vi "log analysis_gps.vi"() -> ()   [LabVIEW 2018] (continued)
\t\n15:44:38.5\tlog_raw\tgps_raw\t\tsystem status\tnormal 2 27.900000 0 0\trobot status\t150.631494\t124.442843\t7.927600\t-0.100159\t-0.498264\t-179.473329\t0.268000\t-0.011000\n\t\n15:44:39.0\tlog_raw\tgps_raw\t\tsystem status\tnormal 2 27.900000 0 0\trobot status\t150.478452\t124.453463\t7.927100\t-0.269341\t-0.623918\t-179.511393\t0.246000\t0.046000\n\t\n15:44:39.5\tlog_raw\tgps_raw\t\tsystem status\tnormal 2 27.900000 0 0\trobot status\t150.333282\t124.462585\t7.928600\t-0.322841\t-0.681958\t-179.469049\t0.260000\t0.066000\n\t\n15:44:40.0\tlog_raw\tgps_raw\t\tsystem status\tnormal 2 27.900000 0 0\trobot status\t150.188702\t124.473109\t7.929800\t-0.268389\t-0.694858\t-179.390159\t0.304000\t0.005000\n\t\n15:44:40.5\tlog_raw\tgps_raw\t\tsystem status\tnormal 2 27.800000 0 0\trobot status\t150.046673\t124.482305\t7.929800\t-0.234085\t-0.771225\t-179.316552\t0.299000\t0.006000\n\t\n15:44:41.0\tlog_raw\tgps_raw\t\tsystem status\tnormal 2 27.900000 0 0\trobot status\t149.902023\t124.492124\t7.930600\t-0.171880\t-0.860108\t-179.202739\t0.268000\t0.042000\n\t\n15:44:41.5\tlog_raw\tgps_raw\t\tsystem status\tnormal 2 27.800000 0 0\trobot status\t149.758940\t124.501657\t7.931700\t-0.049577\t-0.856104\t-179.098606\t0.422000\t-0.186000\n\t\n15:44:42.0\tlog_raw\tgps_raw\t#INSPVAXA,USB3,0,49.5,FINESTEERING,2107,283500.050,02000000,471d,15824;INS_ALIGNMENT_COMPLETE,INS_RTKFIXED,37.37125208894,126.72252418884,7.9323,22.3000,0.0457,-0.3130,0.0162,0.019884592,-0.737230354,268.941103131,0.4422,0.2953,0.5719,0.1133,0.0925,0.0782,0.0964,0.1015,5.0570,0f000001,0*24f2188e\n\tsystem status\tnormal 2 27.800000 0 0\trobot status\t149.616272\t124.511447\t7.932300\t0.019885\t-0.737230\t-178.941103\t0.282000\t0.036000\n\t\n15:44:42.5\tlog_raw\tgps_raw\t\tsystem status\tnormal 2 27.900000 0 0\trobot status\t149.500042\t124.520050\t7.931800\t0.135214\t-0.708677\t-178.779585\t0.109000\t0.043000\n\t\n15:44:43.0\tlog_raw\tgps_raw\t\tsystem status\tnormal 2 27.900000 0 0\trobot status\t149.355950\t124.527273\t7.930800\t0.129535\t-0.692129\t-178.620902\t0.232000\t0.079000\n\t\n15:44:43.5\tlog_raw\tgps_raw\t\tsystem status\tnormal 2 27.900000 0 0\trobot status\t149.217281\t124.534073\t7.930700\t0.247819\t-0.669048\t-178.512392\t0.338000\t-0.027000\n\t\n15:44:44.1\tlog_raw\tgps_raw\t\tsystem status\tnormal 2 27.900000 0 0\trobot status\t149.075473\t124.540045\t7.931300\t0.217256\t-0.509981\t-178.436963\t0.306000\t0.005000\n\t\n15:44:44.6\tlog_raw\tgps_raw\t\tsystem status\tnormal 2 27.800000 0 0\trobot status\t148.934943\t124.543786\t7.931500\t0.099168\t-0.402207\t-178.296990\t0.326000\t-0.034000\n\t\n15:44:45.1\tlog_raw\tgps_raw\t\tsystem status\tnormal 2 27.800000 0 0\trobot status\t148.793897\t124.549425\t7.932200\t0.131171\t-0.388845\t-178.227976\t0.263000\t0.053000\n\t\n15:44:45.6\tlog_raw\tgps_raw\t\tsystem status\tnormal 2 27.900000 0 0\trobot status\t148.653222\t124.555022\t7.931500\t0.252835\t-0.357965\t-178.170042\t0.368000\t-0.106000\n\t\n15:44:46.1\tlog_raw\tgps_raw\t\tsystem status\tnormal 2 27.900000 0 0\trobot status\t148.511244\t124.560395\t7.931600\t0.240454\t-0.345271\t-178.148997\t0.365000\t-0.109000\n\t\n15:44:46.6\tlog_raw\tgps_raw\t\tsystem status\tnormal 2 27.800000 0 0\trobot status\t148.370007\t124.561874\t7.933900\t-0.038867\t-0.502153\t-178.139470\t0.289000\t0.017000\n\t\n15:44:47.1\tlog_raw\tgps_raw\t\tsystem status\tnormal 2 27.900000 0 0\trobot status\t148.234752\t124.565255\t7.935600\t-0.119013\t-0.587133\t-178.082740\t0.262000\t-0.016000\n\t\n15:44:47.6\tlog_raw\tgps_raw\t\tsystem status\tnormal 2 27.800000 0 0\trobot status\t148.145131\t124.569753\t7.937200\t-0.177448\t-0.292844\t-177.902896\t0.342000\t0.062000\n\t\n15:44:48.1\tlog_raw\tgps_raw\t\tsystem status\tnormal 2 27.900000 0 0\trobot status\t148.008420\t124.573995\t7.938300\t-0.006356\t-0.091938\t-177.926561\t0.275000\t-0.003000\n\t\n15:44:48.6\tlog_raw\tgps_raw\t\tsystem status\tnormal 2 27.900000 0 0\trobot status\t147.862293\t124.576815\t7.938300\t0.010797\t-0.019689\t-178.073343\t0.278000\t0.019000\n\t\n15:44:49.1\tlog_raw\tgps_raw\t\tsystem status\tnormal 2 27.900000 0 0\trobot status\t147.729188\t124.580815\t7.939000\t-0.029685\t0.130111\t-178.108993\t0.304000\t-0.009000\n\t\n15:44:49.6\tlog_raw\tgps_raw\t\tsystem status\tnormal 2 27.900000 0 0\trobot status\t147.592276\t124.583432\t7.941800\t-0.099788\t0.170966\t-178.169157\t0.309000\t-0.006000\n\t\n15:44:50.1\tlog_raw\tgps_raw\t#INSPVAXA,USB3,0,48.5,FINESTEERING,2107,283508.100,02000000,471d,15824;INS_ALIGNMENT_COMPLETE,INS_RTKFIXED,37.37125276901,126.72249960907,7.9453,22.3000,0.0373,-0.2902,0.0053,-0.191217202,-0.027683345,268.229043523,0.4412,0.2949,0.5722,0.1131,0.0925,0.0782,0.0964,0.1013,5.0646,0f000001,0*8b85f82b\n\tsystem status\tnormal 2 27.900000 0 0\trobot status\t147.439036\t124.586963\t7.945300\t-0.191217\t-0.027683\t-178.229044\t0.301000\t-0.004000\n\t\n15:44:50.6\tlog_raw\tgps_raw\t\tsystem status\tnormal 2 27.900000 0 0\trobot status\t147.313297\t124.590519\t7.946400\t-0.139869\t-0.013929\t-178.296761\t0.298000\t-0.006000\n\t\n15:44:51.1\tlog_raw\tgps_raw\t#INSPVAXA,USB3,0,51.0,FINESTEERING,2107,283509.100,02000000,471d,15824;INS_ALIGNMENT_COMPLETE,INS_RTKFIXED,37.37125284410,126.72249644466,7.9470,22.3000,0.0401,-0.2879,-0.0045,-0.106806668,-0.162103067,268.404823616,0.4419,0.2950,0.5723,0.1130,0.0925,0.0782,0.0964,0.1013,5.0643,0f000001,0*7bfc8e45\n\tsystem status\tnormal 2 27.900000 0 0\trobot status\t147.158738\t124.595302\t7.947000\t-0.106807\t-0.162103\t-178.404824\t0.301000\t-0.004000\n\t\n15:44:51.6\tlog_raw\tgps_raw\t\tsystem status\tnormal 2 27.900000 0 0\trobot status\t147.032825\t124.599819\t7.947800\t-0.058595\t-0.300497\t-178.519340\t0.302000\t-0.003000\n\t\n15:44:52.1\tlog_raw\tgps_raw\t\tsystem status\tnormal 2 27.900000 0 0\trobot status\t146.935693\t124.606222\t7.947200\t0.018402\t-0.342096\t-178.435886\t0.265000\t-0.053000\n\t\n15:44:52.6\tlog_raw\tgps_raw\t\tsystem status\tnormal 2 27.900000 0 0\trobot status\t146.775595\t124.607523\t7.947200\t-0.117241\t-0.394741\t-178.589413\t0.321000\t-0.041000\n\t\n15:44:53.1\tlog_raw\tgps_raw\t#INSPVAXA,USB3,0,49.5,FINESTEERING,2107,283511.100,02000000,471d,15824;INS_ALIGNMENT_COMPLETE,INS_RTKFIXED,37.37125297857,126.72249062368,7.9478,22.3000,0.0268,-0.2671,0.0078,-0.192910717,-0.348782343,268.576521671,0.4435,0.2952,0.5725,0.1132,0.0925,0.0782,0.0964,0.1012,5.0632,0f000001,0*b468220b\n\tsystem status\tnormal 2 27.900000 0 0\trobot status\t146.643125\t124.610235\t7.947800\t-0.192911\t-0.348782\t-178.576522\t0.289000\t-0.019000\n\t\n15:44:53.6\tlog_raw\tgps_raw\t\tsystem status\tnormal 2 27.900000 0 0\trobot status\t146.501637\t124.614064\t7.947700\t-0.071913\t-0.322697\t-178.749577\t0.298000\t-0.007000\n\t\n15:44:54.1\tlog_raw\tgps_raw\t#INSPVAXA,USB3,0,46.5,FINESTEERING,2107,283512.100,02000000,471d,15824;INS_ALIGNMENT_COMPLETE,INS_RTKFIXED,37.37125304820,126.72248734658,7.9477,22.3000,0.0144,-0.2984,0.0121,-0.146751568,-0.096737224,268.816557460,0.4452,0.2954,0.5727,0.1133,0.0925,0.0782,0.0964,0.1013,5.0625,0f000001,0*292499ae\n\tsystem status\tnormal 2 27.900000 0 0\trobot status\t146.352845\t124.617968\t7.947700\t-0.146752\t-0.096737\t-178.816557\t0.306000\t0.006000\n\t\n15:44:54.6\tlog_raw\tgps_raw\t#INSPVAXA,USB3,0,46.5,FINESTEERING,2107,283512.600,02000000,471d,15824;INS_ALIGNMENT_COMPLETE,INS_RTKFIXED,37.37125307400,126.72248575305,7.9480,22.3000,0.0122,-0.2749,0.0049,-0.358672753,0.036676838,268.917809450,0.4452,0.2954,0.5727,0.1133,0.0925,0.0782,0.0964,0.1013,5.0625,0f000001,0*09269caa\n\tsystem status\tnormal 2 27.900000 0 0\trobot status\t146.211692\t124.620834\t7.948000\t-0.358673\t0.036677\t-178.917809\t0.296000\t-0.004000\n\t\n15:44:55.1\tlog_raw\tgps_raw\t\tsystem status\tnormal 2 27.900000 0 0\trobot status\t146.080792\t124.623760\t7.947900\t-0.500734\t0.107504\t-179.034616\t0.296000\t-0.003000\n\t\n15:44:55.6\tlog_raw\tgps_raw\t\tsystem status\tnormal 2 27.900000 0 0\trobot status\t145.941875\t124.628534\t7.948000\t-0.533837\t0.131507\t-179.099176\t0.299000\t0.000000\n\t\n15:44:56.1\tlog_raw\tgps_raw\t\tsystem status\tnormal 2 27.900000 0 0\trobot status\t145.802261\t124.634287\t7.948900\t-0.548226\t0.140549\t-179.167826\t0.300000\t-0.002000\n\t\n15:44:56.6\tlog_raw\tgps_raw\t\tsystem status\tnormal 2 27.900000 0 0\trobot status\t145.663385\t124.642656\t7.949000\t-0.592979\t-0.128506\t-179.213932\t0.148000\t0.018000\n\t\n15:44:57.1\tlog_raw\tgps_raw\t\tsystem status\tnormal 2 27.800000 0 0\trobot status\t145.577746\t124.651687\t7.948600\t-0.583585\t-0.125120\t-179.114339\t0.350000\t0.047000\n\t\n15:44:57.6\tlog_raw\tgps_raw\t\tsystem status\tnormal 2 27.900000 0 0\trobot status\t145.399589\t124.657796\t7.947700\t-0.657699\t-0.498657\t-179.343167\t0.272000\t0.019000\n\t\n15:44:58.1\tlog_raw\tgps_raw\t#INSPVAXA,USB3,0,46.0,FINESTEERING,2107,283516.100,02000000,471d,15824;INS_ALIGNMENT_COMPLETE,INS_RTKFIXED,37.37125347923,126.72247506393,7.9472,22.3000,0.0170,-0.3545,-0.0054,-0.698217493,-0.526151709,269.397858351,0.4451,0.2957,0.5732,0.1136,0.0925,0.0782,0.0963,0.1013,5.0659,0f000001,0*b20fee82\n\tsystem status\tnormal 2 27.800000 0 0\trobot status\t145.264868\t124.665825\t7.947200\t-0.698217\t-0.526152\t-179.397858\t0.311000\t0.015000\n\t\n15:44:58.6\tlog_raw\tgps_raw\t\tsystem status\tnormal 2 27.900000 0 0\trobot status\t145.120868\t124.672886\t7.946700\t-0.698968\t-0.760852\t-179.547331\t0.292000\t0.004000\n\t\n15:44:59.1\tlog_raw\tgps_raw\t#INSPVAXA,USB3,0,52.0,FINESTEERING,2107,283517.100,02000000,471d,15824;INS_ALIGNMENT_COMPLETE,INS_RTKFIXED,37.37125363028,126.72247167466,7.9449,22.3000,0.0243,-0.3135,0.0010,-0.686347073,-0.797841284,269.600362862,0.4443,0.2956,0.5732,0.1135,0.0925,0.0782,0.0963,0.1013,5.0669,0f000001,0*80e32c69\n\tsystem status\tnormal 2 27.900000 0 0\trobot status\t144.964652\t124.682594\t7.944900\t-0.686347\t-0.797841\t-179.600363\t0.315000\t0.000000\n\t\n15:44:59.6\tlog_raw\tgps_raw\t\tsystem status\tnormal 2 27.900000 0 0\trobot status\t144.838880\t124.691376\t7.944400\t-0.566112\t-0.739210\t-179.635847\t0.288000\t-0.001000\n\t\n15:45:00.1\tlog_raw\tgps_raw\t\tsystem status\tnormal 2 27.900000 0 0\trobot status\t144.692090\t124.700615\t7.944700\t-0.547013\t-0.597270\t-179.727134\t0.296000\t0.005000\n\t\n15:45:00.6\tlog_raw\tgps_raw\t#INSPVAXA,USB3,0,49.0,FINESTEERING,2107,283518.600,02000000,471d,15824;INS_ALIGNMENT_COMPLETE,INS_RTKFIXED,37.37125389857,126.72246679519,7.9445,22.3000,0.0331,-0.3036,0.0138,-0.450567847,-0.447424519,269.738401914,0.4438,0.2956,0.5732,0.1134,0.0925,0.0782,0.0963,0.1013,5.0679,0f000001,0*e0521a7f\n\tsystem status\tnormal 2 27.900000 0 0\trobot status\t144.532436\t124.712378\t7.944500\t-0.450568\t-0.447425\t-179.738402\t0.306000\t0.009000\n\t\n15:45:01.1\tlog_raw\tgps_raw\t\tsystem status\tnormal 2 27.900000 0 0\trobot status\t144.402361\t124.721254\t7.944400\t-0.605900\t-0.247307\t-179.812526\t0.286000\t-0.015000\n\t\n15:45:01.6\tlog_raw\tgps_raw\t\tsystem status\tnormal 2 27.800000 0 0\trobot status\t144.307793\t124.732072\t7.945200\t-0.557084\t-0.001971\t-179.605860\t0.321000\t0.030000\n\t\n15:45:02.1\tlog_raw\tgps_raw\t#INSPVAXA,USB3,0,48.0,FINESTEERING,2107,283520.100,02000000,471d,15824;INS_ALIGNMENT_COMPLETE,INS_RTKFIXED,37.37125419691,126.72246226393,7.9458,22.3000,0.0272,-0.1971,0.0083,-0.453121577,-0.197375891,269.782721447,0.4440,0.2956,0.5733,0.1137,0.0925,0.0782,0.0963,0.1013,5.0706,0f000001,0*56a37df9\n\tsystem status\tnormal 2 27.900000 0 0\trobot status\t144.131065\t124.745496\t7.945800\t-0.453122\t-0.197376\t-179.782721\t0.241000\t0.083000\n\t\n15:45:02.6\tlog_raw\tgps_raw\t#INSPVAXA,USB3,0,51.0,FINESTEERING,2107,283520.600,02000000,471d,15824;INS_ALIGNMENT_COMPLETE,INS_RTKFIXED,37.37125430556,126.72246059927,7.9481,22.3000,0.0288,-0.2781,0.0031,-0.463416060,-0.290924424,269.736679663,0.4440,0.2956,0.5733,0.1137,0.0925,0.0782,0.0963,0.1013,5.0706,0f000001,0*484206e1\n\tsystem status\tnormal 2 27.900000 0 0\trobot status\t143.983612\t124.757557\t7.948100\t-0.463416\t-0.290924\t-179.736680\t0.260000\t0.074000\n\t\n15:45:03.1\tlog_raw\tgps_raw\t\tsystem status\tnormal 2 27.800000 0 0\trobot status\t143.858446\t124.769127\t7.950000\t-0.373602\t-0.343041\t-179.624970\t0.393000\t-0.117000\n\t\n15:45:03.6\tlog_raw\tgps_raw\t\tsystem status\tnormal 2 27.900000 0 0\trobot status\t143.714422\t124.779252\t7.952600\t-0.516012\t-0.390078\t-179.534175\t0.262000\t0.064000\n\t\n15:45:04.1\tlog_raw\tgps_raw\t#INSPVAXA,USB3,0,50.0,FINESTEERING,2107,283522.100,02000000,471d,15824;INS_ALIGNMENT_COMPLETE,INS_RTKFIXED,37.37125461142,126.72245575598,7.9554,22.3000,0.0322,-0.2902,-0.0060,-0.575699494,-0.254956238,269.403721782,0.4439,0.2957,0.5734,0.1134,0.0925,0.0782,0.0963,0.1013,5.0736,0f000001,0*4d3ff4ec\n\tsystem status\tnormal 2 27.800000 0 0\trobot status\t143.554601\t124.791510\t7.955400\t-0.575699\t-0.254956\t-179.403722\t0.286000\t0.027000\n\t\n15:45:04.6\tlog_raw\tgps_raw\t#INSPVAXA,USB3,0,50.0,FINESTEERING,2107,283522.600,02000000,471d,15824;INS_ALIGNMENT_COMPLETE,INS_RTKFIXED,37.37125471396,126.72245415918,7.9561,22.3000,0.0355,-0.2916,-0.0127,-0.527584053,-0.253715800,269.126606548,0.4439,0.2957,0.5734,0.1134,0.0925,0.0782,0.0963,0.1013,5.0736,0f000001,0*ec5fc995\n\tsystem status\tnormal 2 27.800000 0 0\trobot status\t143.413159\t124.802893\t7.956100\t-0.527584\t-0.253716\t-179.126607\t0.295000\t0.016000\n\t\n15:45:05.1\tlog_raw\tgps_raw\t#INSPVAXA,USB3,0,48.5,FINESTEERING,2107,283523.100,02000000,471d,15824;INS_ALIGNMENT_COMPLETE,INS_RTKFIXED,37.37125482190,126.72245252510,7.9566,22.3000,0.0302,-0.2961,-0.0010,-0.338922460,-0.418464715,268.895183147,0.4433,0.2957,0.5734,0.1134,0.0926,0.0782,0.0963,0.1013,5.0752,0f000001,0*1d6fb429\n\tsystem status\tnormal 2 27.800000 0 0\trobot status\t143.268415\t124.814875\t7.956600\t-0.338922\t-0.418465\t-178.895183\t0.302000\t0.007000\n\t\n15:45:05.6\tlog_raw\tgps_raw\t#INSPVAXA,USB3,0,48.5,FINESTEERING,2107,283523.600,02000000,471d,15824;INS_ALIGNMENT_COMPLETE,INS_RTKFIXED,37.37125490537,126.72245090226,7.9573,22.3000,0.0299,-0.3022,0.0033,-0.516635552,-0.400593547,268.699996239,0.4433,0.2957,0.5734,0.1134,0.0926,0.0782,0.0963,0.1013,5.0752,0f000001,0*027b4151\n\tsystem status\tnormal 2 27.800000 0 0\trobot status\t143.124666\t124.824141\t7.957300\t-0.516636\t-0.400594\t-178.699996\t0.373000\t-0.101000\n\t\n15:45:06.1\tlog_raw\tgps_raw\t#INSPVAXA,USB3,0,49.5,FINESTEERING,2107,283524.100,02000000,471d,15824;INS_ALIGNMENT_COMPLETE,INS_RTKFIXED,37.37125498193,126.72244929891,7.9584,22.3000,0.0403,-0.2922,0.0032,-0.646627486,-0.365479151,268.410156940,0.4428,0.2959,0.5733,0.1133,0.0925,0.0782,0.0963,0.1013,5.0766,0f000001,0*7811970f\n\tsystem status\tnormal 2 27.800000 0 0\trobot status\t142.982644\t124.832640\t7.958400\t-0.646627\t-0.365479\t-178.410157\t0.376000\t-0.111000\n\t\n15:45:06.6\tlog_raw\tgps_raw\t\tsystem status\tnormal 2 27.800000 0 0\trobot status\t142.855371\t124.839702\t7.959100\t-0.637911\t-0.389706\t-178.125788\t0.419000\t-0.171000\n\t\n15:45:07.1\tlog_raw\tgps_raw\t\tsystem status\tnormal 2 27.800000 0 0\trobot status\t142.714130\t124.849046\t7.959500\t-0.466492\t-0.305331\t-177.961176\t0.297000\t0.007000\n\t\n15:45:07.6\tlog_raw\tgps_raw\t#INSPVAXA,USB3,0,47.5,FINESTEERING,2107,283525.600,02000000,471d,15824;INS_ALIGNMENT_COMPLETE,INS_RTKFIXED,37.37125519906,126.72244452104,7.9610,22.3000,0.0264,-0.2896,0.0115,-0.459568698,-0.292533166,267.670803857,0.4424,0.2958,0.5732,0.1133,0.0925,0.0782,0.0963,0.1013,5.0781,0f000001,0*17724b4e\n\tsystem status\tnormal 2 27.800000 0 0\trobot status\t142.559428\t124.856746\t7.961000\t-0.459569\t-0.292533\t-177.670804\t0.405000\t-0.152000\n\t\n15:45:08.1\tlog_raw\tgps_raw\t#INSPVAXA,USB3,0,47.0,FINESTEERING,2107,283526.100,02008000,471d,15824;INS_ALIGNMENT_COMPLETE,INS_RTKFIXED,37.37125524446,126.72244292133,7.9621,22.3000,0.0343,-0.2757,0.0102,-0.752609295,-0.423876797,267.522844293,0.4423,0.2959,0.5731,0.1133,0.0925,0.0782,0.0963,0.1013,5.0795,0f000001,0*e02a1c85\n\tsystem status\tnormal 2 27.800000 0 0\trobot status\t142.417729\t124.861787\t7.962100\t-0.752609\t-0.423877\t-177.522844\t0.227000\t0.100000\n\t\n15:45:08.6\tlog_raw\tgps_raw\t\tsystem status\tnormal 2 27.800000 0 0\trobot status\t142.289996\t124.866450\t7.964000\t-0.891263\t-0.489713\t-177.486596\t0.339000\t-0.052000\n\t\n15:45:09.1\tlog_raw\tgps_raw\t#INSPVAXA,USB3,0,47.0,FINESTEERING,2107,283527.100,02008000,471d,15824;INS_ALIGNMENT_COMPLETE,INS_RTKFIXED,37.37125535577,126.72243973319,7.9657,22.3000,0.0385,-0.2807,-0.0002,-0.916031014,-0.466994988,267.419817945,0.4418,0.2957,0.5731,0.1132,0.0925,0.0782,0.0963,0.1013,5.0811,0f000001,0*de1342cb\n\tsystem status\tnormal 2 27.900000 0 0\trobot status\t142.135329\t124.874145\t7.965700\t-0.916031\t-0.466995\t-177.419818\t0.306000\t-0.017000\n\t\n15:45:09.6\tlog_raw\tgps_raw\t#INSPVAXA,USB3,0,48.0,FINESTEERING,2107,283527.600,02008000,471d,15824;INS_ALIGNMENT_COMPLETE,INS_RTKFIXED,37.37125539878,126.72243810634,7.9658,22.3000,0.0326,-0.2757,-0.0036,-1.071635503,-0.660283197,267.417863682,0.4418,0.2957,0.5731,0.1132,0.0925,0.0782,0.0963,0.1013,5.0811,0f000001,0*715093d1\n\tsystem status\tnormal 2 27.900000 0 0\trobot status\t141.991225\t124.878921\t7.965800\t-1.071636\t-0.660283\t-177.417864\t0.236000\t0.079000\n\t\n15:45:10.1\tlog_raw\tgps_raw\t#INSPVAXA,USB3,0,46.5,FINESTEERING,2107,283528.100,02008000,471d,15824;INS_ALIGNMENT_COMPLETE,INS_RTKFIXED,37.37125544077,126.72243647488,7.9658,22.3000,0.0284,-0.2919,-0.0061,-1.262244823,-0.886371740,267.477769914,0.4412,0.2955,0.5730,0.1131,0.0925,0.0782,0.0963,0.1013,5.0826,0f000001,0*a5d2d267\n\tsystem status\tnormal 2 27.900000 0 0\trobot status\t141.846713\t124.883584\t7.965800\t-1.262245\t-0.886372\t-177.477770\t0.371000\t-0.108000\n\t\n15:45:10.6\tlog_raw\tgps_raw\t\tsystem status\tnormal 2 27.900000 0 0\trobot status\t141.737271\t124.888134\t7.965800\t-1.358773\t-1.011232\t-177.503415\t0.249000\t-0.023000\n\t\n15:45:11.1\tlog_raw\tgps_raw\t#INSPVAXA,USB3,0,51.5,FINESTEERING,2107,283529.100,02008000,471d,15824;INS_ALIGNMENT_COMPLETE,INS_RTKFIXED,37.37125551038,126.72243332814,7.9661,22.3000,0.0230,-0.2496,0.0003,-1.593217414,-1.364879356,267.511520433,0.4406,0.2953,0.5729,0.1132,0.0926,0.0782,0.0963,0.1012,5.0841,0f000001,0*c5d25f23\n\tsystem status\tnormal 2 27.900000 0 0\trobot status\t141.567980\t124.891314\t7.966100\t-1.593217\t-1.364879\t-177.511520\t0.254000\t0.059000\n\t\n15:45:11.6\tlog_raw\tgps_raw\t#INSPVAXA,USB3,0,51.5,FINESTEERING,2107,283529.600,02008000,471d,15824;INS_ALIGNMENT_COMPLETE,INS_RTKFIXED,37.37125553545,126.72243179074,7.9678,22.3000,0.0177,-0.3268,0.0196,-1.900322132,-1.296600351,267.646844528,0.4406,0.2953,0.5729,0.1132,0.0926,0.0782,0.0963,0.1012,5.0841,0f000001,0*bf0a8b51\n\tsystem status\tnormal 2 27.900000 0 0\trobot status\t141.431799\t124.894099\t7.967800\t-1.900322\t-1.296600\t-177.646845\t0.334000\t-0.025000\n\t\n15:45:12.1\tlog_raw\tgps_raw\t#INSPVAXA,USB3,0,51.0,FINESTEERING,2107,283530.100,02008000,471d,15824;INS_ALIGNMENT_COMPLETE,INS_RTKFIXED,37.37125556979,126.72243022543,7.9689,22.3000,0.0347,-0.2712,0.0165,-2.106253221,-1.191638715,267.711415615,0.4397,0.2950,0.5729,0.1130,0.0929,0.0782,0.0963,0.1012,5.0852,0f000001,0*30fd5459\n\tsystem status\tnormal 2 27.900000 0 0\trobot status\t141.293147\t124.897913\t7.968900\t-2.106253\t-1.191639\t-177.711416\t0.278000\t0.006000\n\t\n15:45:12.6\tlog_raw\tgps_raw\t#INSPVAXA,USB3,0,51.0,FINESTEERING,2107,283530.600,02000000,471d,15824;INS_ALIGNMENT_COMPLETE,INS_RTKFIXED,37.37125561825,126.72242855799,7.9691,22.3000,0.0407,-0.2688,0.0120,-2.213736166,-1.038882938,267.844151397,0.4397,0.2950,0.5729,0.1130,0.0929,0.0782,0.0963,0.1012,5.0852,0f000001,0*ed713259\n\tsystem status\tnormal 2 27.900000 0 0\trobot status\t141.145448\t124.903293\t7.969100\t-2.213736\t-1.038883\t-177.844151\t0.287000\t0.006000\n\t\n15:45:13.1\tlog_raw\tgps_raw\t#INSPVAXA,USB3,0,43.5,FINESTEERING,2107,283531.100,02000000,471d,15824;INS_ALIGNMENT_COMPLETE,INS_RTKFIXED,37.37125567803,126.72242699713,7.9701,22.3000,0.0384,-0.2967,0.0169,-2.258821559,-0.728124735,267.962573337,0.4398,0.2947,0.5728,0.1130,0.0928,0.0782,0.0963,0.1012,5.0855,0f000001,0*96bde39a\n\tsystem status\tnormal 2 27.900000 0 0\trobot status\t141.007189\t124.909930\t7.970100\t-2.258822\t-0.728125\t-177.962573\t0.307000\t-0.007000\n\t\n15:45:13.6\tlog_raw\tgps_raw\t#INSPVAXA,USB3,0,43.5,FINESTEERING,2107,283531.600,02000000,471d,15824;INS_ALIGNMENT_COMPLETE,INS_RTKFIXED,37.37125573053,126.72242543109,7.9712,22.3000,0.0393,-0.2946,0.0161,-2.393557008,-0.508805819,268.092577363,0.4398,0.2947,0.5728,0.1130,0.0928,0.0782,0.0963,0.1012,5.0855,0f000001,0*fb176aea\n\tsystem status\tnormal 2 27.900000 0 0\trobot status\t140.868472\t124.915759\t7.971200\t-2.393557\t-0.508806\t-178.092577\t0.301000\t-0.006000\n\t\n15:45:14.1\tlog_raw\tgps_raw\t\tsystem status\tnormal 2 27.900000 0 0\trobot status\t140.736365\t124.922041\t7.972000\t-2.497682\t-0.394077\t-178.262431\t0.297000\t-0.011000\n\t\n15:45:14.6\tlog_raw\tgps_raw\t#INSPVAXA,USB3,0,46.5,FINESTEERING,2107,283532.600,02000000,471d,15824;INS_ALIGNMENT_COMPLETE,INS_RTKFIXED,37.37125585668,126.72242215627,7.9725,22.3000,0.0380,-0.3002,0.0167,-2.444436463,-0.411927002,268.408506598,0.4408,0.2948,0.5728,0.1133,0.0928,0.0782,0.0963,0.1013,5.0851,0f000001,0*752f38e5\n\tsystem status\tnormal 2 27.900000 0 0\trobot status\t140.578394\t124.929765\t7.972500\t-2.444436\t-0.411927\t-178.408507\t0.303000\t-0.003000\n\t\n15:45:15.1\tlog_raw\tgps_raw\t#INSPVAXA,USB3,0,46.5,FINESTEERING,2107,283533.100,02000000,471d,15824;INS_ALIGNMENT_COMPLETE,INS_RTKFIXED,37.37125592571,126.72242055610,7.9738,22.3000,0.0424,-0.2920,0.0172,-2.420399044,-0.549310631,268.532317727,0.4414,0.2948,0.5728,0.1132,0.0926,0.0782,0.0963,0.1012,5.0840,0f000001,0*330bd1f6\n\tsystem status\tnormal 2 27.900000 0 0\trobot status\t140.436653\t124.937429\t7.973800\t-2.420399\t-0.549311\t-178.532318\t0.296000\t-0.007000\n\t\n15:45:15.6\tlog_raw\tgps_raw\t#INSPVAXA,USB3,0,49.5,FINESTEERING,2107,283533.600,02000000,471d,15824;INS_ALIGNMENT_COMPLETE,INS_RTKFIXED,37.37125599617,126.72241909319,7.9758,22.3000,0.0239,-0.2932,0.0057,-2.389135000,-0.690009705,268.630043000,0.4414,0.2948,0.5728,0.1132,0.0926,0.0782,0.0963,0.1012,5.0840,0f000001,0*946e4f45\n\tsystem status\tnormal 2 27.900000 0 0\trobot status\t140.307071\t124.945251\t7.975800\t-2.389135\t-0.690010\t-178.630043\t0.283000\t-0.023000\n\t\n15:45:16.1\tlog_raw\tgps_raw\t#INSPVAXA,USB3,0,46.5,FINESTEERING,2107,283534.100,02000000,471d,15824;INS_ALIGNMENT_COMPLETE,INS_RTKFIXED,37.37125606459,126.72241729161,7.9768,22.3000,0.0318,-0.3014,0.0051,-2.433419723,-0.928712698,268.813892776,0.4412,0.2949,0.5728,0.1131,0.0925,0.0782,0.0963,0.1012,5.0833,0f000001,0*8f6d80c9\n\tsystem status\tnormal 2 27.900000 0 0\trobot status\t140.147490\t124.952847\t7.976800\t-2.433420\t-0.928713\t-178.813893\t0.294000\t-0.008000\n\t\n15:45:16.6\tlog_raw\tgps_raw\t#INSPVAXA,USB3,0,46.5,FINESTEERING,2107,283534.600,02000000,471d,15824;INS_ALIGNMENT_COMPLETE,INS_RTKFIXED,37.37125615079,126.72241575292,7.9767,22.3000,0.0422,-0.2723,0.0071,-2.318351029,-0.994572866,268.928791382,0.4412,0.2949,0.5728,0.1131,0.0925,0.0782,0.0963,0.1012,5.0833,0f000001,0*09e2fdbf\n\tsystem status\tnormal 2 27.900000 0 0\trobot status\t140.011195\t124.962416\t7.976700\t-2.318351\t-0.994573\t-178.928791\t0.294000\t-0.011000\n\t\n15:45:17.1\tlog_raw\tgps_raw\t#INSPVAXA,USB3,0,46.5,FINESTEERING,2107,283535.100,02000000,471d,15824;INS_ALIGNMENT_COMPLETE,INS_RTKFIXED,37.37125625866,126.72241406717,7.9767,22.3000,0.0424,-0.2966,-0.0053,-2.021295828,-1.106669357,269.086555595,0.4405,0.2950,0.5729,0.1131,0.0926,0.0782,0.0963,0.1012,5.0840,0f000001,0*6efa0b45\n\tsystem status\tnormal 2 27.900000 0 0\trobot status\t139.861874\t124.974391\t7.976700\t-2.021296\t-1.106669\t-179.086556\t0.304000\t-0.001000\n\t\n15:45:17.6\tlog_raw\tgps_raw\t#INSPVAXA,USB3,0,46.5,FINESTEERING,2107,283535.600,02000000,471d,15824;INS_ALIGNMENT_COMPLETE,INS_RTKFIXED,37.37125636363,126.72241247006,7.9775,22.3000,0.0475,-0.2765,0.0068,-1.865554802,-1.007723760,269.206912297,0.4405,0.2950,0.5729,0.1131,0.0926,0.0782,0.0963,0.1012,5.0840,0f000001,0*0c6af5d6\n\tsystem status\tnormal 2 27.900000 0 0\trobot status\t139.720405\t124.986043\t7.977500\t-1.865555\t-1.007724\t-179.206912\t0.298000\t-0.006000\n\t\n15:45:18.1\tlog_raw\tgps_raw\t#INSPVAXA,USB3,0,47.5,FINESTEERING,2107,283536.100,02000000,471d,15824;INS_ALIGNMENT_COMPLETE,INS_RTKFIXED,37.37125647369,126.72241083113,7.9788,22.3000,0.0521,-0.3007,0.0049,-1.790943231,-0.806222731,269.320889615,0.4398,0.2953,0.5729,0.1129,0.0928,0.0782,0.0963,0.1012,5.0856,0f000001,0*d4e8effb\n\tsystem status\tnormal 2 27.900000 0 0\trobot status\t139.575231\t124.998260\t7.978800\t-1.790943\t-0.806223\t-179.320890\t0.302000\t0.001000\n\t\n15:45:18.6\tlog_raw\tgps_raw\t#INSPVAXA,USB3,0,47.5,FINESTEERING,2107,283536.600,02000000,471d,15824;INS_ALIGNMENT_COMPLETE,INS_RTKFIXED,37.37125658130,126.72240921238,7.9784,22.3000,0.0588,-0.2967,0.0032,-1.856879731,-0.578836067,269.400871435,0.4398,0.2953,0.5729,0.1129,0.0928,0.0782,0.0963,0.1012,5.0856,0f000001,0*690b56d4\n\tsystem status\tnormal 2 27.900000 0 0\trobot status\t139.431845\t125.010206\t7.978400\t-1.856880\t-0.578836\t-179.400871\t0.302000\t0.001000\n\t\n15:45:19.1\tlog_raw\tgps_raw\t#INSPVAXA,USB3,0,46.0,FINESTEERING,2107,283537.100,02000000,471d,15824;INS_ALIGNMENT_COMPLETE,INS_RTKFIXED,37.37125671293,126.72240759051,7.9784,22.3000,0.0622,-0.2885,0.0100,-1.691821646,-0.334147317,269.491731881,0.4392,0.2956,0.5729,0.1129,0.0929,0.0782,0.0963,0.1012,5.0866,0f000001,0*9d354d84\n\tsystem status\tnormal 2 27.900000 0 0\trobot status\t139.288183\t125.024817\t7.978400\t-1.691822\t-0.334147\t-179.491732\t0.296000\t0.000000\n\t\n15:45:19.6\tlog_raw\tgps_raw\t#INSPVAXA,USB3,0,46.0,FINESTEERING,2107,283537.600,02000000,471d,15824;INS_ALIGNMENT_COMPLETE,INS_RTKFIXED,37.37125683698,126.72240594411,7.9786,22.3000,0.0572,-0.2873,0.0166,-1.418143186,-0.126899320,269.581521554,0.4392,0.2956,0.5729,0.1129,0.0929,0.0782,0.0963,0.1012,5.0866,0f000001,0*6d004f4c\n\tsystem status\tnormal 2 27.900000 0 0\trobot status\t139.142347\t125.038587\t7.978600\t-1.418143\t-0.126899\t-179.581522\t0.300000\t0.000000\n\t\n15:45:20.1\tlog_raw\tgps_raw\t#INSPVAXA,USB3,0,49.0,FINESTEERING,2107,283538.100,02000000,471d,15824;INS_ALIGNMENT_COMPLETE,INS_RTKFIXED,37.37125695995,126.72240477426,7.9799,22.3000,0.0495,-0.1342,0.0227,-1.319474925,-0.166358731,269.556076061,0.4404,0.2961,0.5730,0.1144,0.0933,0.0783,0.0963,0.1012,5.0866,0f000001,0*5c5cf594\n\tsystem status\tnormal 2 27.900000 0 0\trobot status\t139.038724\t125.052237\t7.979900\t-1.319475\t-0.166359\t-179.556076\t0.240000\t0.032000\n\t\n15:45:20.6\tlog_raw\tgps_raw\t#INSPVAXA,USB3,0,49.0,FINESTEERING,2107,283538.600,02000000,471d,15824;INS_ALIGNMENT_COMPLETE,INS_RTKFIXED,37.37125706097,126.72240298813,7.9830,22.3000,0.0438,-0.2893,0.0273,-1.369512709,-0.160060416,269.600478230,0.4404,0.2961,0.5730,0.1144,0.0933,0.0783,0.0963,0.1012,5.0866,0f000001,0*64f2f597\n\tsystem status\tnormal 2 27.900000 0 0\trobot status\t138.880511\t125.063451\t7.983000\t-1.369513\t-0.160060\t-179.600478\t0.389000\t-0.129000\n\t\n15:45:21.1\tlog_raw\tgps_raw\t#INSPVAXA,USB3,0,51.0,FINESTEERING,2107,283539.100,02000000,471d,15824;INS_ALIGNMENT_COMPLETE,INS_RTKFIXED,37.37125716893,126.72240151116,7.9851,22.3000,0.0349,-0.3370,0.0409,-1.494089497,0.116619175,269.541070998,0.4422,0.2966,0.5733,0.1130,0.0931,0.0783,0.0963,0.1012,5.0845,0f000001,0*15f1df55\n\tsystem status\tnormal 2 27.900000 0 0\trobot status\t138.749684\t125.075435\t7.985100\t-1.494089\t0.116619\t-179.541071\t0.310000\t0.004000\n\t\n15:45:21.6\tlog_raw\tgps_raw\t#INSPVAXA,USB3,0,51.0,FINESTEERING,2107,283539.600,02000000,471d,15824;INS_ALIGNMENT_COMPLETE,INS_RTKFIXED,37.37125727133,126.72239988665,7.9877,22.3000,0.0429,-0.2928,0.0329,-1.461817471,0.138335830,269.463131487,0.4422,0.2966,0.5733,0.1130,0.0931,0.0783,0.0963,0.1012,5.0845,0f000001,0*8c571713\n\tsystem status\tnormal 2 27.800000 0 0\trobot status\t138.605787\t125.086802\t7.987700\t-1.461817\t0.138336\t-179.463131\t0.357000\t-0.088000\n\t\n15:45:22.1\tlog_raw\tgps_raw\t#INSPVAXA,USB3,0,50.0,FINESTEERING,2107,283540.100,02000000,471d,15824;INS_ALIGNMENT_COMPLETE,INS_RTKFIXED,37.37125737761,126.72239824656,7.9900,22.3000,0.0519,-0.2782,0.0221,-1.451094613,0.074238516,269.298675528,0.4419,0.2969,0.5734,0.1130,0.0929,0.0783,0.0963,0.1012,5.0817,0f000001,0*b323d296\n\tsystem status\tnormal 2 27.800000 0 0\trobot status\t138.460511\t125.098600\t7.990000\t-1.451095\t0.074239\t-179.298676\t0.254000\t0.073000\n\t\n15:45:22.6\tlog_raw\tgps_raw\t#INSPVAXA,USB3,0,50.0,FINESTEERING,2107,283540.600,02000000,471d,15824;INS_ALIGNMENT_COMPLETE,INS_RTKFIXED,37.37125746759,126.72239663487,7.9912,22.3000,0.0429,-0.2872,0.0160,-1.425165250,-0.019252695,269.086348976,0.4419,0.2969,0.5734,0.1130,0.0929,0.0783,0.0963,0.1012,5.0817,0f000001,0*88d26abe\n\tsystem status\tnormal 2 27.800000 0 0\trobot status\t138.317750\t125.108589\t7.991200\t-1.425165\t-0.019253\t-179.086349\t0.256000\t0.066000\n\t\n15:45:23.1\tlog_raw\tgps_raw\t#INSPVAXA,USB3,0,47.0,FINESTEERING,2107,283541.100,02000000,471d,15824;INS_ALIGNMENT_COMPLETE,INS_RTKFIXED,37.37125754334,126.72239500157,7.9927,22.3000,0.0440,-0.2830,0.0173,-1.652300860,-0.379493530,268.915877089,0.4417,0.2969,0.5736,0.1129,0.0927,0.0783,0.0963,0.1011,5.0789,0f000001,0*58806b1d\n\tsystem status\tnormal 2 27.800000 0 0\trobot status\t138.173075\t125.116998\t7.992700\t-1.652301\t-0.379494\t-178.915877\t0.359000\t-0.092000\n\t\n15:45:23.6\tlog_raw\tgps_raw\t#INSPVAXA,USB3,0,47.0,FINESTEERING,2107,283541.600,02000000,471d,15824;INS_ALIGNMENT_COMPLETE,INS_RTKFIXED,37.37125761933,126.72239337708,7.9953,22.3000,0.0493,-0.2834,0.0162,-1.785773716,-0.511638678,268.665930676,0.4417,0.2969,0.5736,0.1129,0.0927,0.0783,0.0963,0.1011,5.0789,0f000001,0*bd9c5353\n\tsystem status\tnormal 2 27.800000 0 0\trobot status\t138.029180\t125.125435\t7.995300\t-1.785774\t-0.511639\t-178.665931\t0.226000\t0.111000\n\t\n15:45:24.1\tlog_raw\tgps_raw\t#INSPVAXA,USB3,0,48.5,FINESTEERING,2107,283542.100,02000000,471d,15824;INS_ALIGNMENT_COMPLETE,INS_RTKFIXED,37.37125769665,126.72239177679,7.9980,22.3000,0.0493,-0.2951,0.0235,-1.875048061,-0.540533252,268.386297576,0.4405,0.2966,0.5735,0.1128,0.0925,0.0783,0.0963,0.1011,5.0773,0f000001,0*2be40074\n\tsystem status\tnormal 2 27.800000 0 0\trobot status\t137.887429\t125.134018\t7.998000\t-1.875048\t-0.540533\t-178.386298\t0.288000\t0.029000\n\t\n15:45:24.6\tlog_raw\tgps_raw\t#INSPVAXA,USB3,0,48.5,FINESTEERING,2107,283542.600,02000000,471d,15824;INS_ALIGNMENT_COMPLETE,INS_RTKFIXED,37.37125775872,126.72239016301,7.9996,22.3000,0.0518,-0.3025,0.0218,-1.945640979,-0.365484318,268.174264778,0.4405,0.2966,0.5735,0.1128,0.0925,0.0783,0.0963,0.1011,5.0773,0f000001,0*896be2ff\n\tsystem status\tnormal 2 27.800000 0 0\trobot status\t137.744483\t125.140909\t7.999600\t-1.945641\t-0.365484\t-178.174265\t0.364000\t-0.097000\n\t\n15:45:25.1\tlog_raw\tgps_raw\t#INSPVAXA,USB3,0,47.5,FINESTEERING,2107,283543.100,02000000,471d,15824;INS_ALIGNMENT_COMPLETE,INS_RTKFIXED,37.37125783022,126.72238854441,8.0007,22.3000,0.0360,-0.2808,0.0229,-1.906190638,-0.356725874,267.886535177,0.4398,0.2962,0.5735,0.1128,0.0925,0.0783,0.0963,0.1011,5.0772,0f000001,0*1744d296\n\tsystem status\tnormal 2 27.800000 0 0\trobot status\t137.601110\t125.148847\t8.000700\t-1.906191\t-0.356726\t-177.886535\t0.223000\t0.112000\n\t\n15:45:25.6\tlog_raw\tgps_raw\t#INSPVAXA,USB3,0,47.5,FINESTEERING,2107,283543.600,02000000,471d,15824;INS_ALIGNMENT_COMPLETE,INS_RTKFIXED,37.37125788763,126.72238692132,8.0016,22.3000,0.0356,-0.2896,0.0094,-1.979603347,-0.321373170,267.681718152,0.4398,0.2962,0.5735,0.1128,0.0925,0.0783,0.0963,0.1011,5.0772,0f000001,0*45f837fc\n\tsystem status\tnormal 2 27.800000 0 0\trobot status\t137.457340\t125.155221\t8.001600\t-1.979603\t-0.321373\t-177.681718\t0.198000\t0.144000\n\t\n15:45:26.1\tlog_raw\tgps_raw\t#DUALANTENNAHEADINGA,USB3,0,47.5,FINESTEERING,2107,283544.100,02000000,d426,15824;INSUFFICIENT_OBS,NONE,-1.000000000,0.000000000,0.000000000,0.0,0.000000000,0.000000000,\"631T\",12,4,4,3,04,00,20,02*84d96ce8\n\tsystem status\tnormal 2 27.800000 0 0\trobot status\t137.314501\t125.161172\t8.002300\t-2.139049\t-0.267810\t-177.508872\t0.389000\t-0.146000\n\t\n15:45:26.6\tlog_raw\tgps_raw\t#INSPVAXA,USB3,0,51.0,FINESTEERING,2107,283544.600,02000000,471d,15824;INS_ALIGNMENT_COMPLETE,INS_RTKFIXED,37.37125797814,126.72238366933,8.0025,22.3000,0.0382,-0.2769,0.0143,-2.206615640,-0.357729210,267.363519498,0.4396,0.2961,0.5737,0.1128,0.0924,0.0783,0.0964,0.1011,5.0776,0f000001,0*0a578cde\n\tsystem status\tnormal 2 27.800000 0 0\trobot status\t137.169284\t125.165271\t8.002500\t-2.206616\t-0.357729\t-177.363519\t0.318000\t-0.039000\n\t\n15:45:27.1\tlog_raw\tgps_raw\t#INSPVAXA,USB3,0,49.5,FINESTEERING,2107,283545.100,02000000,471d,15824;INS_ALIGNMENT_COMPLETE,INS_RTKFIXED,37.37125803132,126.72238203676,8.0019,22.3000,0.0517,-0.2764,0.0124,-2.158934023,-0.436592254,267.230007610,0.4389,0.2957,0.5737,0.1127,0.0924,0.0783,0.0964,0.1011,5.0787,0f000001,0*62787010\n\tsystem status\tnormal 2 27.800000 0 0\trobot status\t137.024673\t125.171176\t8.001900\t-2.158934\t-0.436592\t-177.230008\t0.258000\t0.045000\n\t\n15:45:27.6\tlog_raw\tgps_raw\t#INSPVAXA,USB3,0,49.5,FINESTEERING,2107,283545.600,02000000,471d,15824;INS_ALIGNMENT_COMPLETE,INS_RTKFIXED,37.37125808188,126.72238043700,8.0001,22.3000,0.0477,-0.2875,0.0096,-2.125628520,-0.371940065,267.210451376,0.4389,0.2957,0.5737,0.1127,0.0924,0.0783,0.0964,0.1011,5.0787,0f000001,0*6d8598a7\n\tsystem status\tnormal 2 27.900000 0 0\trobot status\t136.882969\t125.176789\t8.000100\t-2.125629\t-0.371940\t-177.210451\t0.246000\t0.069000\n\t\n15:45:28.1\tlog_raw\tgps_raw\t#DUALANTENNAHEADINGA,USB3,0,49.0,FINESTEERING,2107,283546.100,02000000,d426,15824;INSUFFICIENT_OBS,NONE,-1.000000000,0.000000000,0.000000000,0.0,0.000000000,0.000000000,\"631T\",14,4,4,3,04,00,20,03*f6e7f028\n\tsystem status\tnormal 2 27.900000 0 0\trobot status\t136.739120\t125.182335\t7.997800\t-2.208188\t-0.262010\t-177.222030\t0.282000\t0.016000\n\t\n15:45:28.6\tlog_raw\tgps_raw\t#INSPVAXA,USB3,0,49.0,FINESTEERING,2107,283546.600,02000000,471d,15824;INS_ALIGNMENT_COMPLETE,INS_RTKFIXED,37.37125815693,126.72237718708,7.9959,22.3000,0.0472,-0.2869,0.0097,-2.448876962,-0.301078601,267.272161666,0.4388,0.2955,0.5737,0.1127,0.0924,0.0783,0.0964,0.1011,5.0802,0f000001,0*b5ddd59b\n\tsystem status\tnormal 2 27.900000 0 0\trobot status\t136.595097\t125.185123\t7.995900\t-2.448877\t-0.301079\t-177.272162\t0.283000\t0.003000\n\t\n15:45:29.1\tlog_raw\tgps_raw\t#DUALANTENNAHEADINGA,USB3,0,49.0,FINESTEERING,2107,283547.100,02000000,d426,15824;INSUFFICIENT_OBS,NONE,-1.000000000,0.000000000,0.000000000,0.0,0.000000000,0.000000000,\"631T\",13,4,4,3,04,00,20,03*d1017fba\n\tsystem status\tnormal 2 27.900000 0 0\trobot status\t136.452881\t125.189037\t7.994800\t-2.629921\t-0.272001\t-177.284144\t0.314000\t-0.013000\n\t\n15:45:29.6\tlog_raw\tgps_raw\t#DUALANTENNAHEADINGA,USB3,0,50.5,FINESTEERING,2107,283547.600,02000000,d426,15824;INSUFFICIENT_OBS,NONE,-1.000000000,0.000000000,0.000000000,0.0,0.000000000,0.000000000,\"631T\",14,4,4,3,04,00,20,03*23b2448a\n\tsystem status\tnormal 2 27.800000 0 0\trobot status\t136.339828\t125.193852\t7.993700\t-2.593766\t-0.035037\t-177.075383\t0.326000\t0.039000\n\t\n15:45:30.1\tlog_raw\tgps_raw\t#INSPVAXA,USB3,0,48.5,FINESTEERING,2107,283548.100,02000000,471d,15824;INS_ALIGNMENT_COMPLETE,INS_RTKFIXED,37.37125826747,126.72237261641,7.9908,22.3000,0.0551,-0.2062,0.0107,-2.709225073,-0.117327049,267.249046746,0.4386,0.2951,0.5737,0.1130,0.0926,0.0783,0.0964,0.1011,5.0831,0f000001,0*59a87063\n\tsystem status\tnormal 2 27.900000 0 0\trobot status\t136.190234\t125.197398\t7.990800\t-2.709225\t-0.117327\t-177.249047\t0.239000\t0.049000\n\t\n15:45:30.6\tlog_raw\tgps_raw\t#INSPVAXA,USB3,0,48.5,FINESTEERING,2107,283548.600,02000000,471d,15824;INS_ALIGNMENT_COMPLETE,INS_RTKFIXED,37.37125828182,126.72237093999,7.9873,22.3000,0.0467,-0.3123,0.0115,-2.842538161,-0.073425539,267.267184569,0.4386,0.2951,0.5737,0.1130,0.0926,0.0783,0.0964,0.1011,5.0831,0f000001,0*3db09e30\n\tsystem status\tnormal 2 27.900000 0 0\trobot status\t136.041740\t125.198993\t7.987300\t-2.842538\t-0.073426\t-177.267185\t0.319000\t-0.026000\n\t\n15:45:31.1\tlog_raw\tgps_raw\t#INSPVAXA,USB3,0,49.0,FINESTEERING,2107,283549.100,02000000,471d,15824;INS_ALIGNMENT_COMPLETE,INS_RTKFIXED,37.37125831392,126.72236948257,7.9859,22.3000,0.0458,-0.3107,0.0117,-2.935659020,0.110600359,267.341322191,0.4389,0.2949,0.5737,0.1127,0.0927,0.0783,0.0964,0.1010,5.0837,0f000001,0*651f733f\n\tsystem status\tnormal 2 27.900000 0 0\trobot status\t135.912644\t125.202558\t7.985900\t-2.935659\t0.110600\t-177.341322\t0.300000\t-0.003000\n\t\n15:45:31.6\tlog_raw\tgps_raw\t#DUALANTENNAHEADINGA,USB3,0,49.0,FINESTEERING,2107,283549.600,02000000,d426,15824;INSUFFICIENT_OBS,NONE,-1.000000000,0.000000000,0.000000000,0.0,0.000000000,0.000000000,\"631T\",12,4,4,3,04,00,20,03*a5c8d3a9\n\tsystem status\tnormal 2 27.900000 0 0\trobot status\t135.766974\t125.205952\t7.986800\t-2.944950\t0.268420\t-177.447000\t0.294000\t-0.013000\n\t\n15:45:32.1\tlog_raw\tgps_raw\t#INSPVAXA,USB3,0,49.0,FINESTEERING,2107,283550.100,02000000,471d,15824;INS_ALIGNMENT_COMPLETE,INS_RTKFIXED,37.37125837980,126.72236622244,7.9865,22.3000,0.0464,-0.2979,0.0062,-2.970555166,0.308033741,267.553888887,0.4387,0.2947,0.5737,0.1126,0.0926,0.0783,0.0963,0.1010,5.0837,0f000001,0*d140be5a\n\tsystem status\tnormal 2 27.900000 0 0\trobot status\t135.623867\t125.209874\t7.986500\t-2.970555\t0.308034\t-177.553889\t0.303000\t0.004000\n\t\n15:45:32.6\tlog_raw\tgps_raw\t#INSPVAXA,USB3,0,50.5,FINESTEERING,2107,283550.600,02000000,471d,15824;INS_ALIGNMENT_COMPLETE,INS_RTKFIXED,37.37125841199,126.72236465933,7.9851,22.3000,0.0388,-0.2917,0.0030,-2.826015531,0.302597414,267.642559027,0.4387,0.2947,0.5737,0.1126,0.0926,0.0783,0.0963,0.1010,5.0837,0f000001,0*d1068808\n\tsystem status\tnormal 2 27.900000 0 0\trobot status\t135.485409\t125.213449\t7.985100\t-2.826016\t0.302597\t-177.642559\t0.302000\t-0.003000\n\t\n15:45:33.1\tlog_raw\tgps_raw\t#DUALANTENNAHEADINGA,USB3,0,46.5,FINESTEERING,2107,283551.100,02000000,d426,15824;INSUFFICIENT_OBS,NONE,-1.000000000,0.000000000,0.000000000,0.0,0.000000000,0.000000000,\"631T\",12,4,4,3,04,00,20,03*69312952\n\tsystem status\tnormal 2 27.900000 0 0\trobot status\t135.345730\t125.216481\t7.983600\t-2.721815\t0.236235\t-177.735291\t0.301000\t-0.007000\n\t\n15:45:33.6\tlog_raw\tgps_raw\t#INSPVAXA,USB3,0,46.5,FINESTEERING,2107,283551.600,02000000,471d,15824;INS_ALIGNMENT_COMPLETE,INS_RTKFIXED,37.37125843948,126.72236147331,7.9829,22.3000,0.0386,-0.2728,0.0018,-2.861657525,0.138389194,267.863675039,0.4385,0.2948,0.5738,0.1126,0.0925,0.0783,0.0963,0.1010,5.0836,0f000001,0*5dcd711b\n\tsystem status\tnormal 2 27.900000 0 0\trobot status\t135.203197\t125.216505\t7.982900\t-2.861658\t0.138389\t-177.863675\t0.296000\t-0.009000\n\t\n15:45:34.1\tlog_raw\tgps_raw\t#DUALANTENNAHEADINGA,USB3,0,44.5,FINESTEERING,2107,283552.100,02000000,d426,15824;INSUFFICIENT_OBS,NONE,-1.000000000,0.000000000,0.000000000,0.0,0.000000000,0.000000000,\"631T\",13,4,4,3,04,00,20,03*c0320929\n\tsystem status\tnormal 2 27.900000 0 0\trobot status\t135.076743\t125.216703\t7.982100\t-3.027561\t-0.013602\t-177.989904\t0.291000\t-0.016000\n\t\n15:45:34.6\tlog_raw\tgps_raw\t#DUALANTENNAHEADINGA,USB3,0,44.5,FINESTEERING,2107,283552.600,02000000,d426,15824;INSUFFICIENT_OBS,NONE,-1.000000000,0.000000000,0.000000000,0.0,0.000000000,0.000000000,\"631T\",14,4,4,3,04,00,20,03*46a498f4\n\tsystem status\tnormal 2 27.900000 0 0\trobot status\t134.938712\t125.217325\t7.982200\t-2.950461\t-0.123683\t-178.092242\t0.300000\t-0.002000\n\t\n15:45:35.1\tlog_raw\tgps_raw\t#DUALANTENNAHEADINGA,USB3,0,44.5,FINESTEERING,2107,283553.100,02000000,d426,15824;INSUFFICIENT_OBS,NONE,-1.000000000,0.000000000,0.000000000,0.0,0.000000000,0.000000000,\"631T\",13,4,4,3,04,00,20,03*adea0df0\n
